vi "TA_Plot_SelectedKinetics_3.vi"(8 "Selected\nWavelength (nm)":dbl[](array[numeric])=[432.0, 534.0, 643.0], 9 "File Path":path=path "/Users/tm/Desktop/fs-TA/Data/demo_fsta.dat") -> (2 "TA Selected Kinetics":cluster{"Array":dbl[], "Array 2":dbl[]}[](graph), 3 "Selected Kinetics":dbl[][](array[numeric]))   [LabVIEW 2025]
uses:
  TA_DATA.ctl
panel:
  out "TA Data":T1
  out "Actual Selected Wavelength":dbl[](array[numeric])
  out "DeltaA for Selected Wavelength":dbl[][](array[numeric])
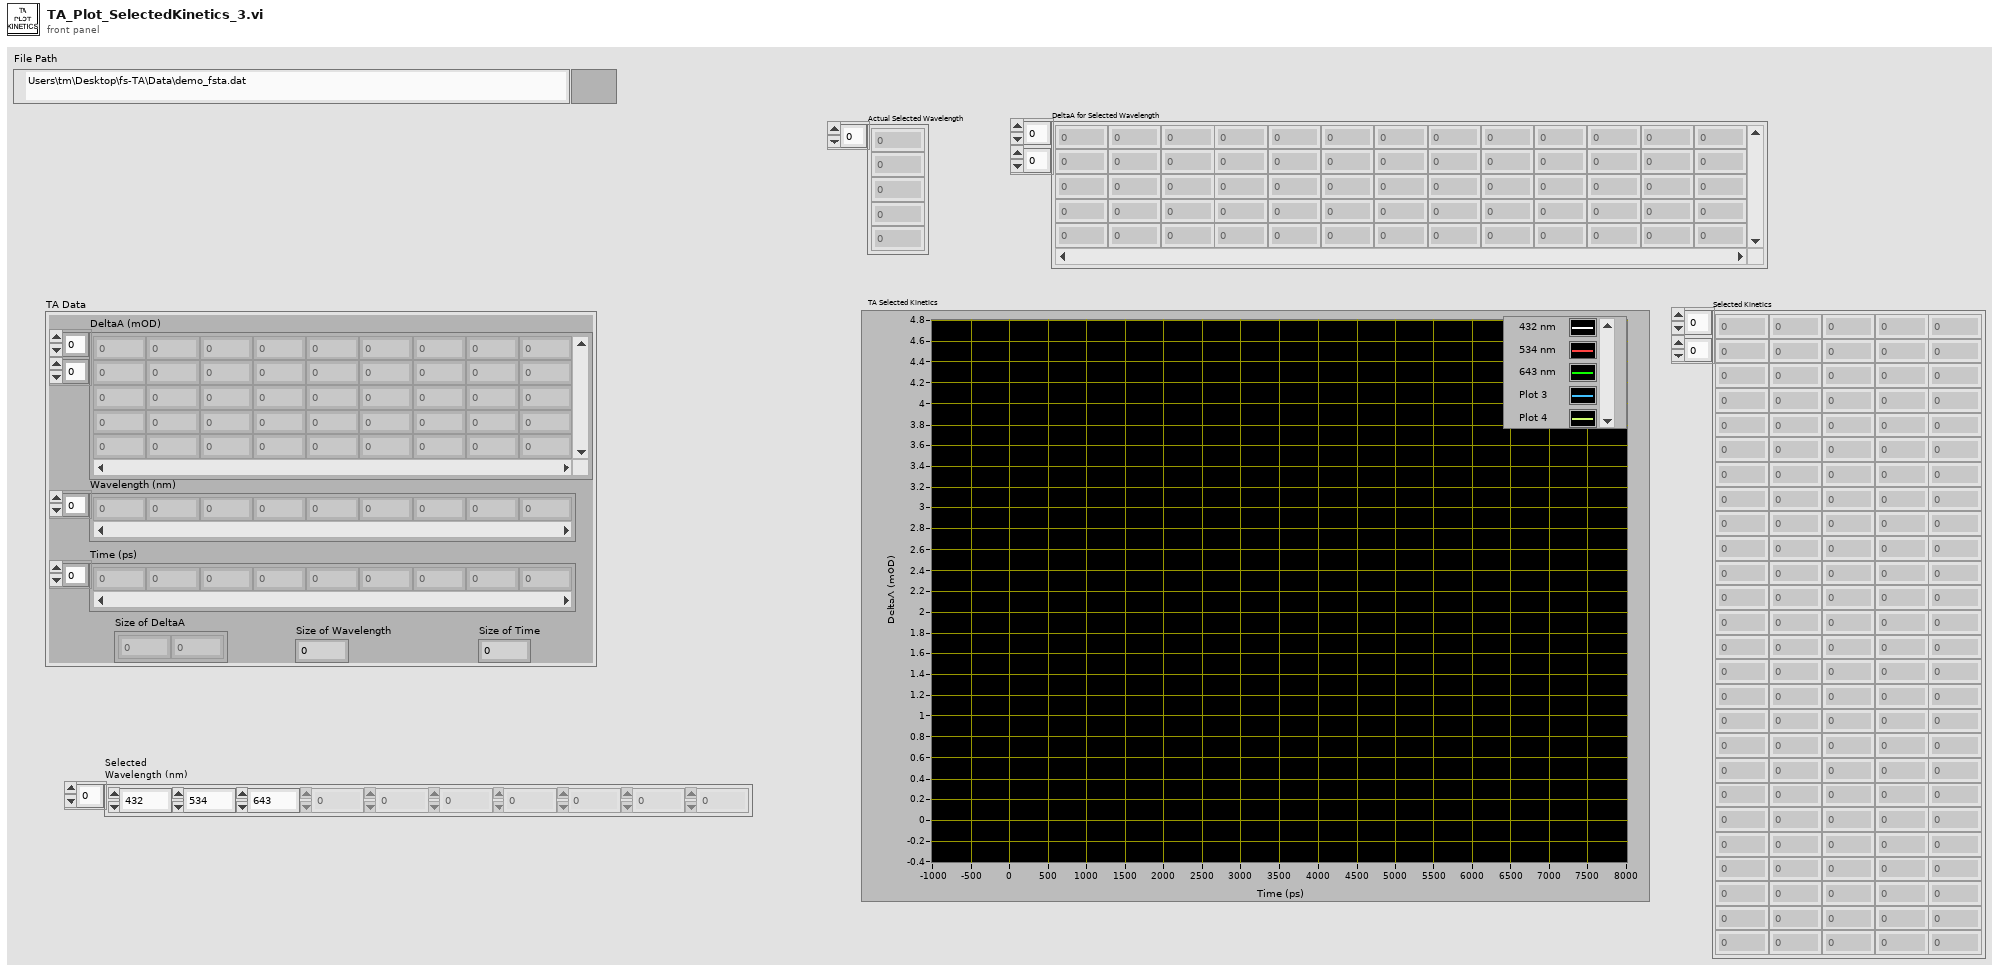
[diagram p1: front panel]
types:
  T1 = typedef "TA_DATA.ctl" = cluster{"DeltaA (mOD)":dbl[][], "Wavelength (nm)":dbl[], "Time (ps)":dbl[], "Size of DeltaA":i32[], "Size of Wavelength":i32, "Size of Time":i32}
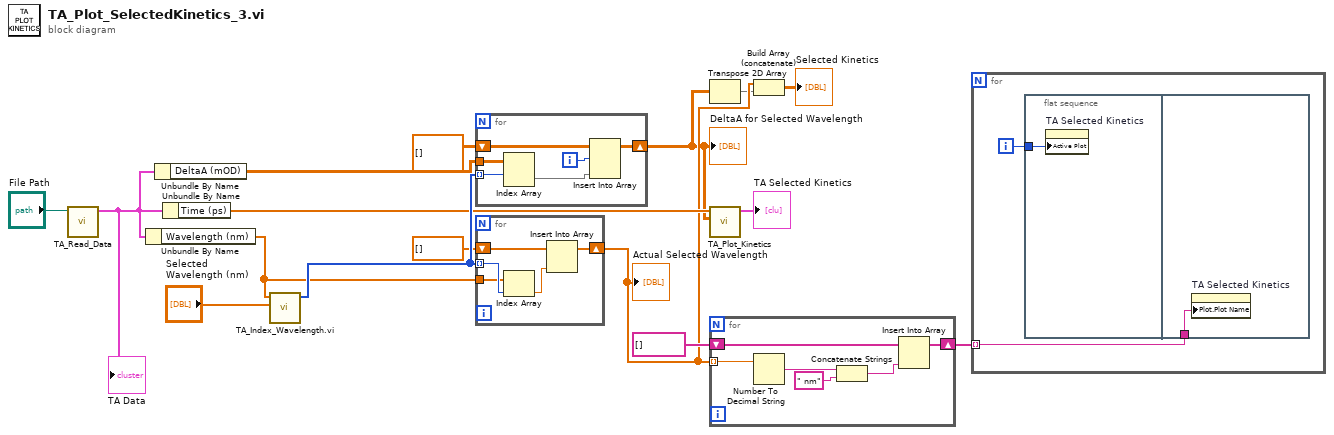
[diagram p0: block diagram]
diagram:
  n1 = call "TA_Read_Data.vi"("File Path"="File Path") -> ("TA Data"=w1:T1)  [unwired: 10 in]
  "TA Data" <- w1
  n2 = Unbundle By Name(w1) -> ("Wavelength (nm)"=w10:dbl[])
  n3 = Unbundle By Name(w1) -> ("DeltaA (mOD)"=w9:dbl[][])
  n4 = Unbundle By Name(w1) -> ("Time (ps)"=w13:dbl[])
  n5 = call "TA_Index_Wavelength.vi.vi"("Selected Wavelength"="Selected\nWavelength (nm)", "Wavelength (nm)"=w10) -> ("Index of Selected Wavelength"=w14:i32[])  [unwired: 9 in]
  n6 = for {
    shift-right: [w20] -> w4
    shift-left: dbl[][] [] ("Array") -> [w22]
    tunnel: w14 -> [w19] mode=indexing
    tunnel: w9 -> [w17]
    i -> [w18]
    n7 = Index Array(array=w17, index (row)=w19) -> (element=w21:dbl[])  [unwired: 1 in]
    n8 = Insert Into Array(array=w22, index (row)=w18, new element=w21) -> (w20:dbl[][])  [unwired: 1 in]
  }
  "DeltaA for Selected Wavelength" <- w4
  n9 = for {
    shift-right: [w26] -> w5
    shift-left: dbl[] [] ("Array") -> [w25]
    tunnel: w14 -> [w27] mode=indexing
    tunnel: w10 -> [w24]
    n10 = Index Array(array=w24, index=w27) -> (element=w23:dbl)
    n11 = Insert Into Array(array=w25, new element=w23) -> (w26:dbl[])  [unwired: 1 in]
  }
  "Actual Selected Wavelength" <- w5
  n12 = Transpose 2D Array(2D array=w4) -> (transposed array=w3:dbl[][])
  n13 = call "TA_Plot_Kinetics.vi"("DeltaA (mOD)"=w4, "Time (ps)"=w13) -> ("TA Kinetics"=→"TA Selected Kinetics":cluster{"Array":dbl[], "Array 2":dbl[]}[])  [unwired: 9 in]
  n14 = for {
    tunnel: w5 -> [w33] mode=indexing
    shift-right: [w28] -> w7
    shift-left: string[] [] ("Array") -> [w29]
    n15 = Number To Decimal String(number=w33) -> (decimal integer string=w31:string)  [unwired: 1 in]
    n16 = Concatenate Strings(w31, " nm" ("string")) -> (w30:string)
    n17 = Insert Into Array(array=w29, new element=w30) -> (w28:string[])  [unwired: 1 in]
  }
  n18 = Build Array (concatenate)(w5, w3) -> (→"Selected Kinetics":dbl[][])
  n19 = for {
    tunnel: w7 -> [w35] mode=indexing
    i -> [w34]
    n20 = flat-sequence {
      tunnel: w34 -> [w36]
      tunnel: w35 -> [w37]
      frame #0 {
        n21 = property on="TA Selected Kinetics" class="XYGraph (strict)"("Active Plot"=w36) -> ()  [unwired: 2 in, 2 out]
      }
      frame #1 {
        n22 = property on="TA Selected Kinetics" class="XYGraph (strict)"("Plot.Plot Name"=w37) -> ()  [unwired: 2 in, 2 out]
      }
    }
  }
